vi "gun.vi"() -> ()   [LabVIEW 2011]
uses:
  common/scale_const.ctl
  common/gain_const.ctl
  common/gain_bin_sched_const.ctl
  gun_motor_state.ctl
  <vilib>/Rock Robotics/SystemInterfaces/Typedef/FPGA_TypedefDigitalModule.ctl
  <vilib>/Rock Robotics/SystemInterfaces/DIO/FPGA_DIOChannel.ctl
  signals/Signal.ctl
  <vilib>/Rock Robotics/WPI/Relay/WPI_RelayValue.ctl
  gun_tracking_mode.ctl
  Robot Global Data.vi
  Program Files (x86)/National Instruments/LabVIEW 2011/examples/FRC/I2C/HiTechnic Compass/Driver/HiTechnic Compass.lvlib
panel:
  in  "gun speed const":T1={"min_ana"=0.0, "min_units"=2200.0, "max_ana"=1.0, "max_units"=2200.0}
  in  "fender speed const":T1={"min_ana"=0.0, "min_units"=1650.0, "max_ana"=1.0, "max_units"=1730.0}
  in  "light time":u32=150
  in  "Gains Fender":T2={"Positive"={"kP"=1.4, "kI"=3.3, "kD"=0.06}, "Netative"={"kP"=1.4, "kI"=3.3, "kD"=0.06}}
  in  "Gains Key":T2={"Positive"={"kP"=1.45, "kI"=3.5, "kD"=0.057}, "Netative"={"kP"=1.5, "kI"=3.3, "kD"=0.054}}
  in  "PID Fender":T3={"kP"=1.0, "kI"=3.0, "kD"=0.06}
  in  "interval back key":dbl=1000.0
  in  "interval fender":dbl=1000.0
  in  "interval key":dbl=650.0
  in  "Cam Lock Const":u32=150
  in  "Hood Key":dbl=67.0
  in  "Gun Key":dbl=2200.0
  in  "back key Gun":dbl=2200.0
  in  "back key Hood":dbl=68.0
  in  "Scale Const":T1={"min_ana"=0.0, "min_units"=90.0, "max_ana"=25.5, "max_units"=82.5}
  out "Heading":dbl
  # "Fender Shot"
  # "Key Shot"
  # "Back Key Shot"
  # "kP 1.5\nkI 3.3\nkD .054"
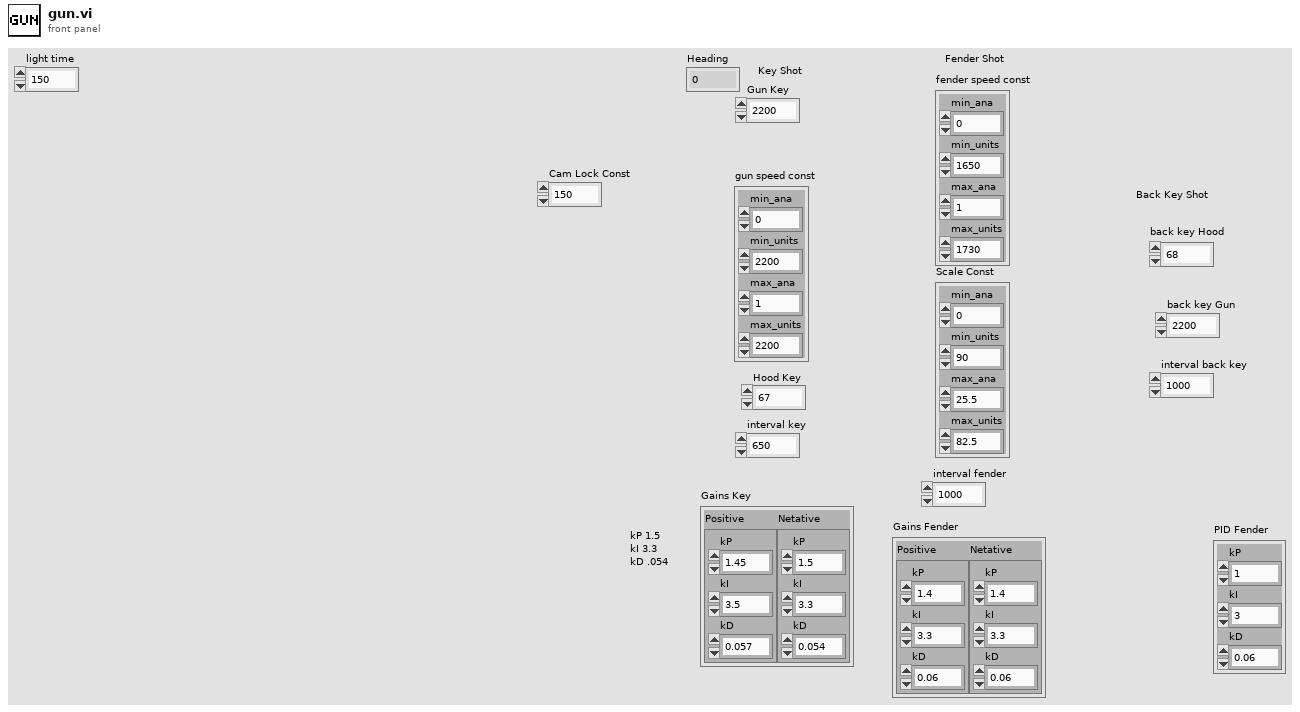
[diagram p1: front panel]
types:
  T1 = typedef "scale_const.ctl" = cluster{"min_ana":dbl, "min_units":dbl, "max_ana":dbl, "max_units":dbl}
  T2 = typedef "gain_bin_sched_const.ctl" = cluster{"Positive":cluster{"kP":dbl, "kI":dbl, "kD":dbl}, "Netative":cluster{"kP":dbl, "kI":dbl, "kD":dbl}}
  T3 = typedef "gain_const.ctl" = cluster{"kP":dbl, "kI":dbl, "kD":dbl}
  T4 = typedef "FPGA_DIOChannel.ctl" = enum8{"DIO 1", "DIO 2", "DIO 3", "DIO 4", "DIO 5", "DIO 6", "DIO 7", "DIO 8", "DIO 9", "DIO 10", "DIO 11", "DIO 12", "DIO 13", "DIO 14", "Invalid"}
  T5 = typedef "FPGA_TypedefDigitalModule.ctl" = enum16{"Digital Module 1", "Digital Module 2"}
  T6 = typedef "gun_motor_state.ctl" = enum16{"Hold Power", "Hold Speed", "Hold Distance", "Stop"}
  T7 = cluster{"Gun Key":dbl, "Shooter Control Mode":T6}
  T8 = typedef "WPI_DigitalInputDevRef.ctl" = cluster{"DevStatus":errorcluster, "DIO Channel":T4, "Digital Module":T5}
  T9 = typedef "WPI_I2CDevRef.ctl" = cluster{"DevStatus":errorcluster, "Digital Module":T5, "Device Address":u8}
  T10 = typedef "WPI_RelayDevRef.ctl" = cluster{"DevStatus":errorcluster, "Relay Channel":T11, "Digital Module":T5, "Relay Direction":T12}
  T11 = typedef "FPGA_DIORelayChannel.ctl" = enum8{"Relay 1", "Relay 2", "Relay 3", "Relay 4", "Relay 5", "Relay 6", "Relay 7", "Relay 8", "Invalid"}
  T12 = typedef "WPI_RelayDirection.ctl" = enum16{"Both directions", "Forward only", "Reverse only"}
  T13 = typedef "Signal.ctl" = enum16{"SIGFIRE", "SIGSTOPSCRIPT", "SIGSTARTGUN", "SIGSTOPGUN", "SIGDISABLED", "SIGENABLED", "SIGUDPTIMEOUT", "SIGNEWVISION_REMOTE", "SIGNEWVISION_LOCAL", "SIGSHOTFIRED", "SIGDOTRACK", "SIGDONTTRACK"}
  T14 = typedef "WPI_RelayValue.ctl" = enum16{"Off", "On", "Forward", "Reverse"}
  T15 = typedef "gun_tracking_mode.ctl" = enum16{"manual_aim", "auto_aim_camera", "preset_center_field", "preset_right_pocket", "preset_left_pocket", "align_center", "align_center_backwards", "auto_aim_key", "align_fold", "auton_custom", "preset_pass", "auto_aim_auton"}
  T16 = typedef "gun_rt_fast_upstream_data.ctl" = cluster{"gun_sensor_speed":dbl, "gun_motor_output":dbl}
  T17 = typedef "gun_rt_slow_upstream_data.ctl" = cluster{"turret":cluster{"turret_analog":dbl, "turret_angle":dbl, "turret_motor":dbl, "turret_idg_state":T18}, "hood":cluster{"hood_analog":dbl, "hood_angle":dbl, "hood_motor":dbl, "hood_idg_state":T18}}
  T18 = typedef "idg_trust_t.ctl" = enum16{"fault_move", "fault_high", "fault_low", "out_high", "out_low", "trust"}
  T19 = typedef "user_data.ctl" = cluster{"Driver":cluster{"Buttons":T20, "Axes":cluster{"L-X":dbl, "L-Y":dbl, "R-X":dbl, "R-Y":dbl, "D-X":dbl, "D-Y":dbl}}, "Operator":cluster{"Buttons":T21, "Axes":cluster{"L-X":dbl, "L-Y":dbl, "Trig":dbl, "R-X":dbl, "R-Y":dbl, "D-X":dbl}}, "Kittys Kat Box":cluster{"Btn1":bool, "Btn2":bool, "Btn3":bool, "LeftKnob":dbl, "RightKnob":dbl, "SW1":bool, "SW2":bool}}
  T20 = typedef "user_buttons_dualaction.ctl" = cluster{"Btn1":bool, "Btn2":bool, "Btn3":bool, "Btn4":bool, "L1":bool, "R1":bool, "L2":bool, "R2":bool, "Face-L":bool, "Face-R":bool, "L3":bool, "R3":bool}
  T21 = typedef "user_buttons_360.ctl" = cluster{"Down":bool, "Right":bool, "Left":bool, "Up":bool, "L1":bool, "R1":bool, "Face-L":bool, "Face-R":bool, "L2":bool, "R2":bool, "Unused":bool, "Unused":bool}
  T22 = typedef "gun_rt_slow_downstream_data.ctl" = cluster{"turret":cluster{"turret_setpoint":dbl, "turret_reset_integral":bool, "turret_manual":dbl, "turret_manual_mode":bool}, "hood":cluster{"hood_setpoint":dbl, "hood_reset_integral":bool, "hood_manual":dbl, "hood_manual_mode":bool}}
  T23 = typedef "gun_preset_pos_t.ctl" = enum16{"Center Field", "Right Pocket", "Left Pocket", "Align Center", "Align Center Backwards", "Fold Side", "Pass"}
  T24 = typedef "gun_preset_bundle_t.ctl" = cluster{"speed":dbl, "turret":dbl, "hood":dbl, "interval":dbl}
  T25 = cluster{"speed":dbl, "hood":dbl, "speed new":dbl}
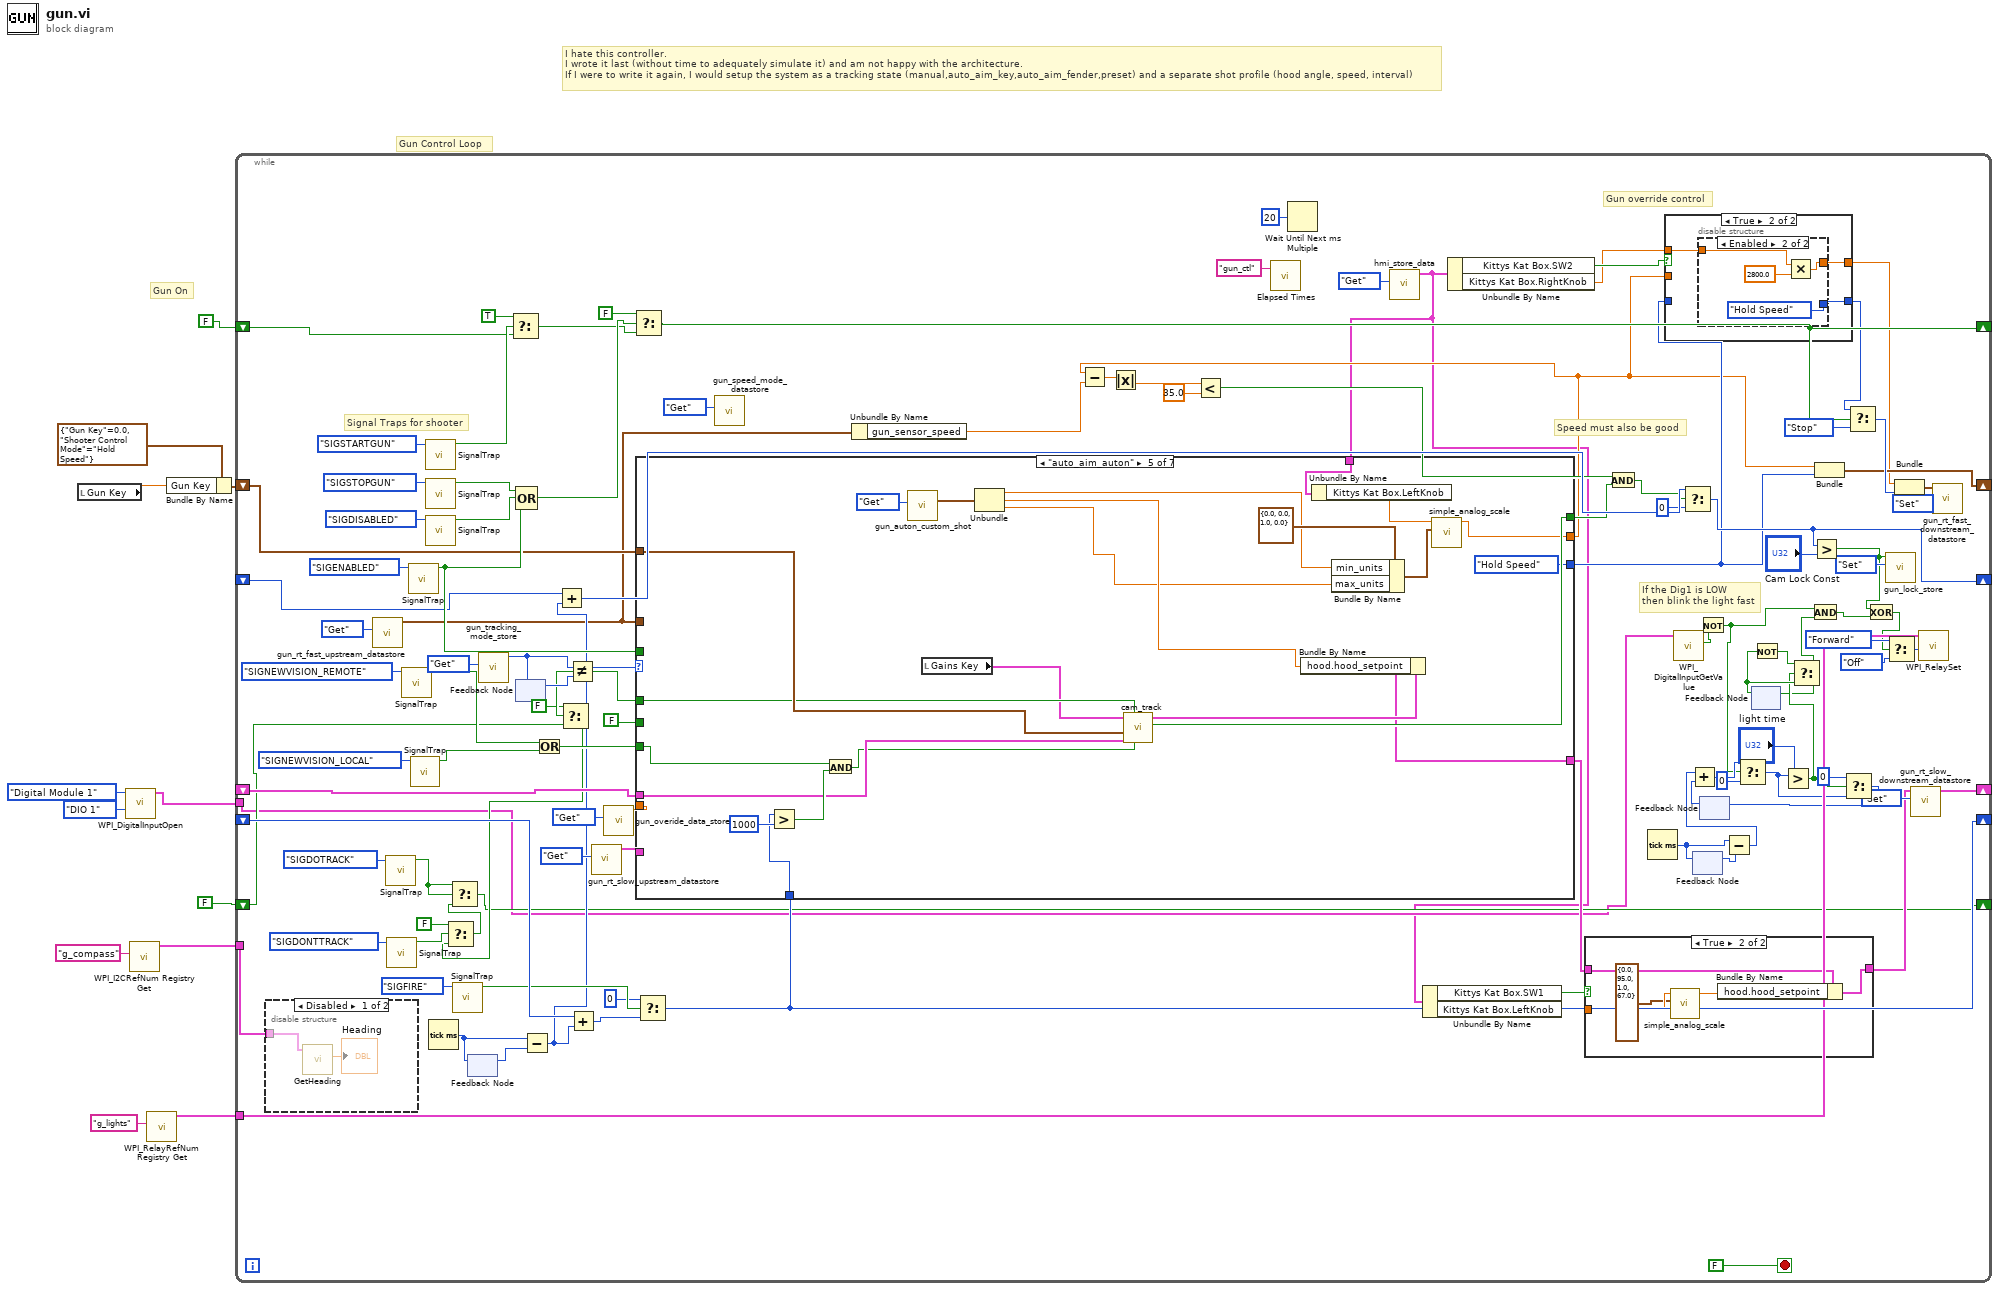
[diagram p0: block diagram]
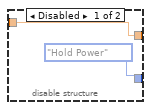
[diagram p4: hidden frame]
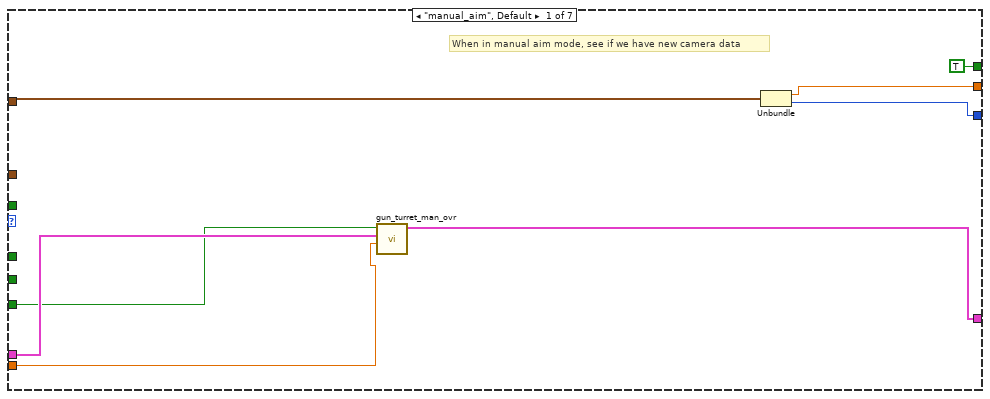
[diagram p6: hidden frame]
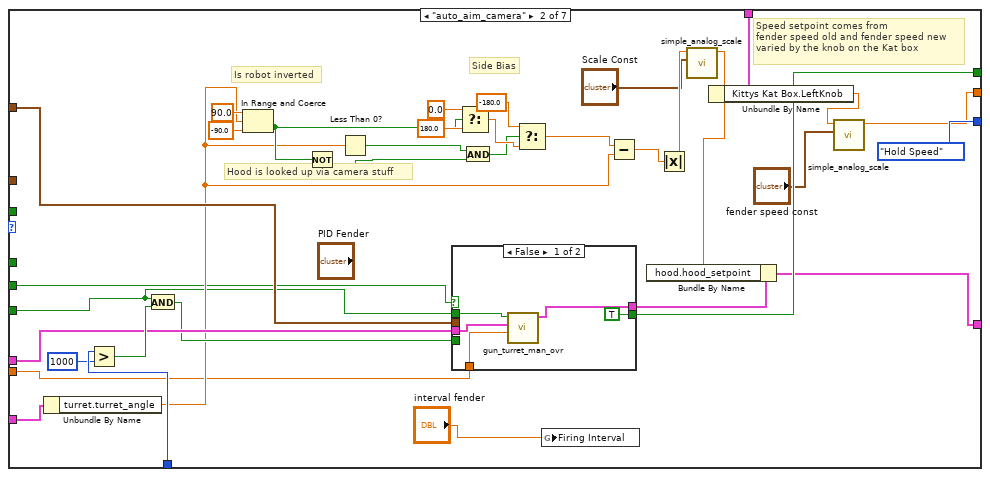
[diagram p7: hidden frame]
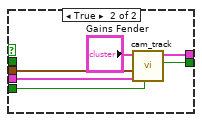
[diagram p8: hidden frame]
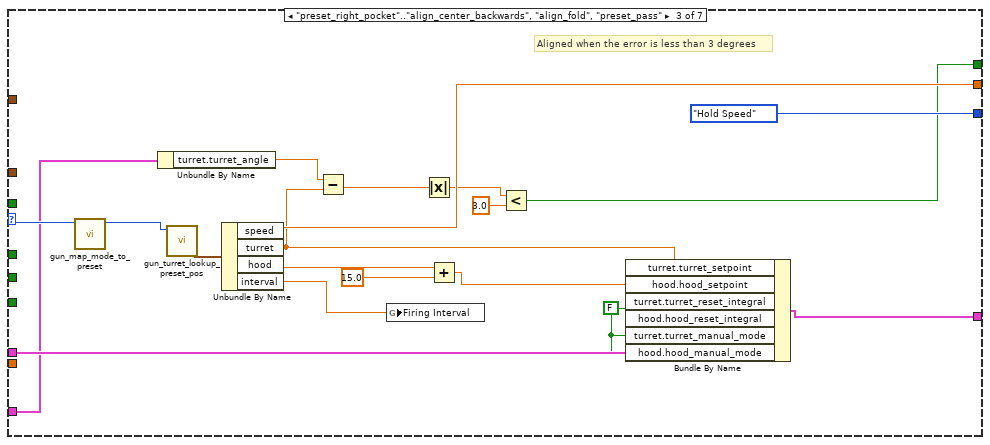
[diagram p9: hidden frame]
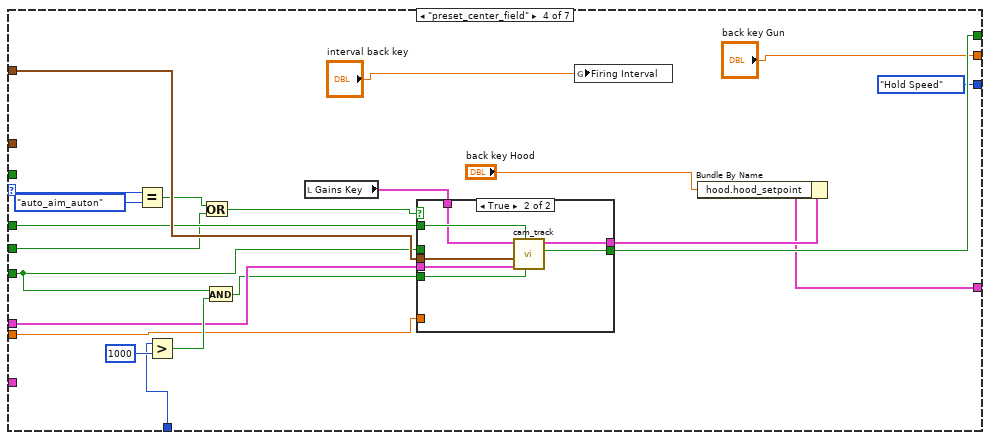
[diagram p10: hidden frame]
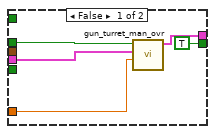
[diagram p11: hidden frame]
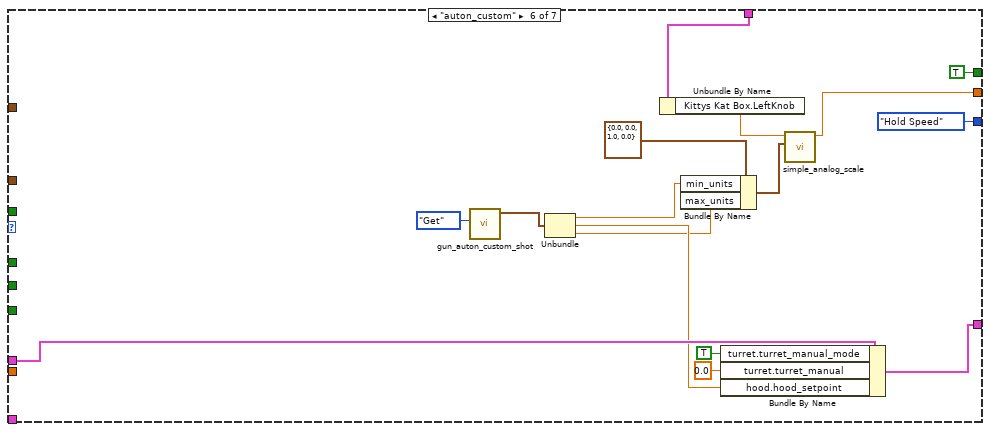
[diagram p12: hidden frame]
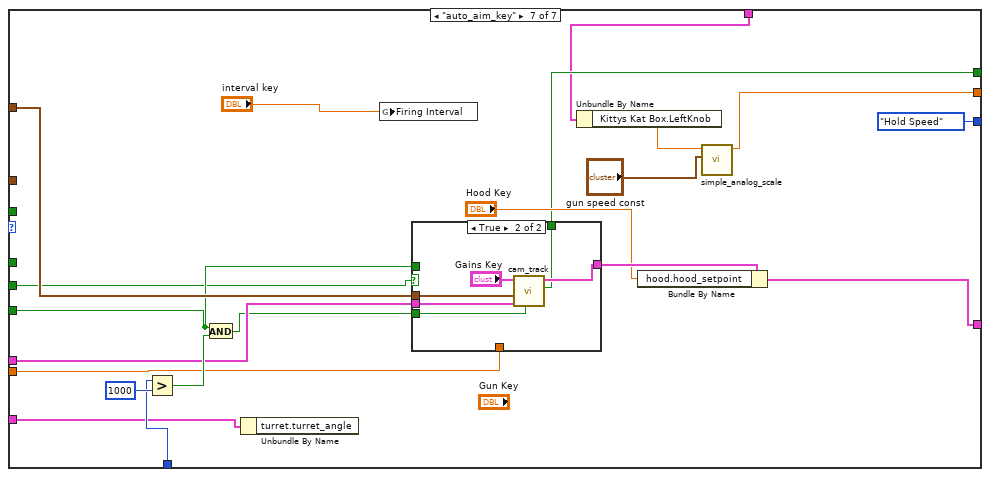
[diagram p13: hidden frame]
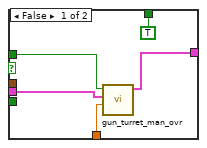
[diagram p14: hidden frame]
diagram:
  # "I hate this controller.\nI wrote it last (without time to adequately simulate it) and am not happy with the architecture.\nIf I were to write it again, I would setup the system as a tracking state (manual,auto_aim_key,auto_aim_fender,preset) and a separate shot profile (hood angle, speed, interval)"
  # "Gun On"
  # "Gun Control Loop"
  n1 = local read "Gun Key"() -> (w5:dbl)
  n2 = call <vilib>:"WPI_DigitalInputOpen.vi"("DIO Channel"=FPGA_DIOChannel."DIO 1", "Digital Module (Module 1)"=FPGA_TypedefDigitalModule."Digital Module 1") -> ("DigitalInputDevRef"=w3:T8)  [unwired: 8 in, 1 out]
  n3 = call <vilib>:"WPI_I2CRefNum Registry Get.vi"("refnum name"="g_compass") -> ("I2CDevRef"=w10:T9)  [unwired: 9 in, 1 out]
  n4 = call <vilib>:"WPI_RelayRefNum Registry Get.vi"("refnum name"="g_lights") -> ("RelayDevRef"=w8:T10)  [unwired: 9 in, 1 out]
  n5 = Bundle By Name(cluster=T7 {"Gun Key"=0.0, "Shooter Control Mode"=enum."Hold Speed"}, "Gun Key"=w5) -> (w6:T7)
  n6 = while {
    shift-right: [w90] -> _
    shift-left: FALSE -> [w120]
    shift-right: [w97] -> _
    shift-left: _ -> [w89]
    shift-right: [w79] -> _
    shift-left: w6 -> [w65]
    tunnel: w10 -> [w88]
    shift-right: [w80] -> _
    shift-left: _ -> [w84]
    shift-right: [w71] -> _
    shift-left: _ -> [w75]
    tunnel: w8 -> [w60]
    shift-right: [w35] -> _
    shift-left: FALSE -> [w36]
    tunnel: w3 -> [w31]
    stop <- FALSE stop-if-true
    # "If the Dig1 is LOW\nthen blink the light fast"
    # "Gun override control"
    # "Speed must also be good"
    # "Signal Traps for shooter"
    n7 = disable-structure shown="Disabled" {
      disable-tunnel: w88 -> [w143 _]
      frame Disabled {
        n8 = call "GetHeading.vi"("I2CDevRef"=w143) -> ("Heading"=→"Heading":dbl)  [unwired: 1 in, 9 out]
      }
      frame Enabled {
      }
    }
    n9 = call "gun_rt_fast_upstream_datastore.vi"("data_store_mode"=enum16{"Set", "Get"}."Get") -> ("gun_rt_fast_upstream_data out"=w64:T16)  [unwired: 10 in]
    n10 = call "SignalTrap.vi"("Signal"=Signal."SIGDOTRACK") -> ("Trapped Signal"=w44:bool)  [unwired: 10 in]
    n11 = call "SignalTrap.vi"("Signal"=Signal."SIGDONTTRACK") -> ("Trapped Signal"=w40:bool)  [unwired: 10 in]
    n12 = call "SignalTrap.vi"("Signal"=Signal."SIGNEWVISION_REMOTE") -> ("Trapped Signal"=w95:bool)  [unwired: 10 in]
    n13 = call "SignalTrap.vi"("Signal"=Signal."SIGENABLED") -> ("Trapped Signal"=w91:bool)  [unwired: 10 in]
    n14 = call "SignalTrap.vi"("Signal"=Signal."SIGNEWVISION_LOCAL") -> ("Trapped Signal"=w94:bool)  [unwired: 10 in]
    n15 = call "SignalTrap.vi"("Signal"=Signal."SIGSTARTGUN") -> ("Trapped Signal"=w121:bool)  [unwired: 10 in]
    n16 = call "SignalTrap.vi"("Signal"=Signal."SIGSTOPGUN") -> ("Trapped Signal"=w118:bool)  [unwired: 10 in]
    n17 = call "SignalTrap.vi"("Signal"=Signal."SIGDISABLED") -> ("Trapped Signal"=w117:bool)  [unwired: 10 in]
    n18 = Tick Count (ms)() -> (millisecond timer value=w85:u32)
    n19 = call "SignalTrap.vi"("Signal"=Signal."SIGFIRE") -> ("Trapped Signal"=w82:bool)  [unwired: 10 in]
    n20 = feedback-in #1(w85) -> ()
    n21 = feedback #1() -> (w86:u32)  [unwired: 1 in]
    n22 = call "gun_tracking_mode_store.vi"("data_store_mode"=enum16{"Set", "Get"}."Get") -> ("gun tracking mode"=w76:T15)  [unwired: 10 in]
    n23 = Select(t=TRUE, s=w121, f=w120) -> (s? t:f=w111:bool)
    n24 = Compound Arithmetic op=OR(w118, w117, w91) -> (w116:bool)
    n25 = feedback-in #2(w76) -> ()
    n26 = feedback #2() -> (w77:T15)  [unwired: 1 in]
    n27 = Subtract(x=w85, y=w86) -> (x-y=w74:u32)
    n28 = Or(x=w95, y=w94) -> (x .or. y?=w93:bool)
    n29 = Add(x=w75, y=w74) -> (x+y=w73:u32)
    n30 = Not Equal?(x=w76, y=w77) -> (x != y?=w43:bool)
    n31 = Select(t=FALSE, s=w43, f=w36) -> (s? t:f=w37:bool)
    n32 = Select(t=FALSE, s=w40, f=w37) -> (s? t:f=w39:bool)
    n33 = Select(t=w44, s=w44, f=w39) -> (s? t:f=w35:bool)
    n34 = Add(x=w84, y=w74) -> (x+y=w83:u32)
    n35 = call "gun_rt_slow_upstream_datastore.vi"("data_store_mode"=enum16{"Set", "Get"}."Get") -> ("gun_rt_slow_upstream_data out"=w92:T17)  [unwired: 10 in]
    n36 = call "gun_overide_data_store.vi"("mode"=enum16{"Set", "Get"}."Get") -> ("Overide Out"=w98:dbl)  [unwired: 10 in]
    n37 = Select(t=FALSE, s=w116, f=w111) -> (s? t:f=w90:bool)
    n38 = Select(t=u32 0, s=w82, f=w83) -> (s? t:f=w80:u32)
    n39 = call "gun_speed_mode_datastore.vi"("data_store_mode"=enum16{"Set", "Get"}."Get") -> ()  [unwired: 10 in, 1 out]
    n40 = Unbundle By Name(w64) -> ("gun_sensor_speed"=w66:dbl)
    n41 = call "Elapsed Times.vi"("Call Name"="gun_ctl") -> ()  [unwired: 2 in, 1 out]
    n42 = Wait Until Next ms Multiple(millisecond multiple=u32 20 ("milliseconds to wait")) -> ()  [unwired: 1 out]
    n43 = call "hmi_store_data.vi"("data_store_mode"=enum16{"Set", "Get"}."Get") -> ("UserData out"=w13:T19)  [unwired: 10 in]
    n44 = case shown="\"auto_aim_auton\"" w76 {
      selector: w76 -> [_ _ w216 w221 _ _ _]
      tunnel: [w146 w154 w213 "back key Gun" w253 w278 w291] -> w51
      tunnel: w98 -> [w148 w156 _ w222 _ _ w295]
      tunnel: w89 -> [w151 w167 w212 w235 w270 w287 w304]
      tunnel: w65 -> [w147 w168 _ w234 w269 _ w303]
      tunnel: w93 -> [w149 w157 _ w223 w261 _ w296]
      tunnel: w92 -> [_ w186 w208 _ _ _ w306]
      tunnel: w91 -> [_ _ _ _ _ _ _]
      tunnel: [w150 w164 w211 w229 w265 w284 w299] -> w48
      tunnel: [w145 gun_motor_state."Hold Speed" ("Shooter Control Mode") gun_motor_state."Hold Speed" ("t") gun_motor_state."Hold Speed" ("Shooter Control Mode") gun_motor_state."Hold Speed" ("Shooter Control Mode") gun_motor_state."Hold Speed" ("Shooter Control Mode") gun_motor_state."Hold Speed" ("Shooter Control Mode")] -> w53
      tunnel: w80 -> [_ w185 _ w236 w271 _ w307]
      tunnel: [TRUE ("Lock") w166 w202 w233 w268 TRUE ("Lock") w298] -> w62
      tunnel: w43 -> [_ _ _ w225 w263 _ _]
      tunnel: w64 -> [_ _ _ _ _ _ _]
      tunnel: FALSE ("t") -> [_ w158 _ w218 _ _ w294]
      tunnel: w13 -> [_ w153 _ _ w254 w279 w292]
      frame "manual_aim", Default {
        # "When in manual aim mode, see if we have new camera data"
        n45 = call "gun_turret_man_ovr.vi"("Overide"=w148, "gun_rt_slow_downstream_data out in"=w151, "Trigger Vision"=w149) -> ("gun_rt_slow_downstream_data out out"=w150:T22)  [unwired: 8 in]
        n46 = Unbundle(w147) -> ("Units"=w146:dbl, "Shooter Control Mode"=w145:T6)
      }
      frame "auto_aim_camera" {
        # "Speed setpoint comes from\nfender speed old and fender speed new\nvaried by the knob on the Kat box"
        # "Side Bias"
        # "Is robot inverted"
        # "Hood is looked up via camera stuff"
        n47 = Unbundle By Name(w186) -> ("turret.turret_angle"=w160:dbl)
        n48 = Greater?(x=w185, y=u32 1000) -> (0:w183:bool)
        n49 = And(x=w157, y=w183) -> (x .and. y?=w161:bool)
        n50 = In Range and Coerce(upper limit=90.0, x=w160, lower limit=-90.0) -> (In Range?=w171:bool)  [unwired: 1 out]
        n51 = Not(x=w171) -> (.not. x?=w172:bool)
        n52 = Less Than 0?(x=w160) -> (x < 0?=w174:bool)
        n53 = case shown="False" w158 {
          tunnel: w168 -> [_ w197]
          tunnel: w167 -> [w190 w196]
          tunnel: [TRUE ("Lock") w195] -> w166
          tunnel: [w189 w194] -> w165
          tunnel: w161 -> [_ w193]
          tunnel: w157 -> [w191 _]
          tunnel: w156 -> [w187 _]
          frame False {
            n54 = call "gun_turret_man_ovr.vi"("Overide"=w187, "gun_rt_slow_downstream_data out in"=w190, "Trigger Vision"=w191) -> ("gun_rt_slow_downstream_data out out"=w189:T22)  [unwired: 8 in]
          }
          frame True {
            n55 = call "cam_track.vi"("Trigger"=w193, "gun_rt_slow_downstream_data out in"=w196, "gun_rt_fast_downstream_data out"=w197, "Gains"="Gains Fender") -> ("Lock"=w195:bool, "gun_rt_slow_downstream_data out out"=w194:T22)  [unwired: 6 in]
          }
        }
        n56 = Select(t=0.0, s=w171, f=180.0) -> (s? t:f=w178:dbl)
        n57 = And(x=w174, y=w172) -> (x .and. y?=w173:bool)
        n58 = Select(t=-180.0, s=w173, f=w178) -> (s? t:f=w176:dbl)
        n59 = global write "Robot Global Data.vi" "Firing Interval"("interval fender") -> ()
        n60 = Subtract(x=w176, y=w160) -> (x-y=w175:dbl)
        n61 = Absolute Value(x=w175) -> (abs(x)=w170:dbl)
        n62 = call "simple_analog_scale.vi"("Scale Const"="Scale Const", "Analog"=w170) -> ("Units"=w163:dbl)  [unwired: 9 in]
        n63 = Bundle By Name(cluster=w165, "hood.hood_setpoint"=w163) -> (w164:T22)
        n64 = Unbundle By Name(w153) -> ("Kittys Kat Box.LeftKnob"=w152:dbl)
        n65 = call "simple_analog_scale.vi"("Scale Const"="fender speed const", "Analog"=w152) -> ("Units"=w154:dbl)  [unwired: 9 in]
      }
      frame "preset_right_pocket".."align_center_backwards", "align_fold", "preset_pass" {
        w210 = FALSE
        # "Aligned when the error is less than 3 degrees"
        n66 = call "gun_map_mode_to_preset.vi"("gun tracking mode"=w216) -> ("Preset Position"=w215:T23)  [unwired: 10 in]
        n67 = Unbundle By Name(w208) -> ("turret.turret_angle"=w207:dbl)
        n68 = call "gun_turret_lookup_preset_pos.vi"("Preset Position"=w215) -> ("Position"=w214:T24)  [unwired: 10 in]
        n69 = Unbundle By Name(w214) -> ("speed"=w213:dbl, "turret"=w206:dbl, "hood"=w201:dbl, "interval"=w198:dbl)
        n70 = Subtract(x=w207, y=w206) -> (x-y=w205:dbl)
        n71 = global write "Robot Global Data.vi" "Firing Interval"(w198) -> ()
        n72 = Absolute Value(x=w205) -> (abs(x)=w204:dbl)
        n73 = Add(x=w201, y=15.0) -> (x+y=w200:dbl)
        n74 = Less?(x=w204, y=3.0) -> (x < y?=w202:bool)
        n75 = Bundle By Name(cluster=w212, "turret.turret_setpoint"=w206, "hood.hood_setpoint"=w200, "turret.turret_reset_integral"=w210, "hood.hood_reset_integral"=w210, "turret.turret_manual_mode"=w210, "hood.hood_manual_mode"=w210) -> (w211:T22)
      }
      frame "preset_center_field" {
        n76 = Equal?(x=w221, y=gun_tracking_mode."auto_aim_auton") -> (x = y?=w219:bool)
        n77 = Greater?(x=w236, y=u32 1000) -> (0:w237:bool)
        n78 = Or(x=w219, y=w218) -> (x .or. y?=w217:bool)
        n79 = And(x=w223, y=w237) -> (x .and. y?=w227:bool)
        n80 = local read "Gains Key"() -> (w224:T2)
        n81 = case shown="True" w217 {
          tunnel: w235 -> [w242 w250]
          tunnel: w234 -> [_ w249]
          tunnel: [TRUE ("Lock") w248] -> w233
          tunnel: [w241 w247] -> w230
          tunnel: w227 -> [_ w246]
          tunnel: w225 -> [_ w245]
          tunnel: w224 -> [_ w244]
          tunnel: w223 -> [w243 _]
          tunnel: w222 -> [w239 _]
          frame False {
            n82 = call "gun_turret_man_ovr.vi"("Overide"=w239, "gun_rt_slow_downstream_data out in"=w242, "Trigger Vision"=w243) -> ("gun_rt_slow_downstream_data out out"=w241:T22)  [unwired: 8 in]
          }
          frame True {
            n83 = call "cam_track.vi"("Trigger"=w246, "state change"=w245, "gun_rt_slow_downstream_data out in"=w250, "gun_rt_fast_downstream_data out"=w249, "Gains"=w244) -> ("Lock"=w248:bool, "gun_rt_slow_downstream_data out out"=w247:T22)  [unwired: 5 in]
          }
        }
        n84 = global write "Robot Global Data.vi" "Firing Interval"("interval back key") -> ()
        n85 = Bundle By Name(cluster=w230, "hood.hood_setpoint"="back key Hood") -> (w229:T22)
      }
      frame "auto_aim_auton" {
        n86 = Greater?(x=w271, y=u32 1000) -> (0:w272:bool)
        n87 = And(x=w261, y=w272) -> (x .and. y?=w264:bool)
        n88 = call "gun_auton_custom_shot.vi"("data_store_mode"=enum16{"Set", "Get"}."Get") -> ("shot params out"=w259:T25)  [unwired: 10 in]
        n89 = local read "Gains Key"() -> (w262:T2)
        n90 = Unbundle(w259) -> ("speed"=w252:dbl, "hood"=w258:dbl, "speed new"=w251:dbl)
        n91 = call "cam_track.vi"("Trigger"=w264, "state change"=w263, "gun_rt_slow_downstream_data out in"=w270, "gun_rt_fast_downstream_data out"=w269, "Gains"=w262) -> ("Lock"=w268:bool, "gun_rt_slow_downstream_data out out"=w266:T22)  [unwired: 5 in]
        n92 = Bundle By Name(cluster=w266, "hood.hood_setpoint"=w258) -> (w265:T22)
        n93 = Unbundle By Name(w254) -> ("Kittys Kat Box.LeftKnob"=w257:dbl)
        n94 = Bundle By Name(cluster=T1 {"min_ana"=0.0, "min_units"=0.0, "max_ana"=1.0, "max_units"=0.0} ("Scale Const"), "min_units"=w252, "max_units"=w251) -> (w255:T1)
        n95 = call "simple_analog_scale.vi"("Scale Const"=w255, "Analog"=w257) -> ("Units"=w253:dbl)  [unwired: 9 in]
      }
      frame "auton_custom" {
        n96 = call "gun_auton_custom_shot.vi"("data_store_mode"=enum16{"Set", "Get"}."Get") -> ("shot params out"=w282:T25)  [unwired: 10 in]
        n97 = Unbundle(w282) -> ("speed"=w275:dbl, "hood"=w281:dbl, "speed new"=w274:dbl)
        n98 = Unbundle By Name(w279) -> ("Kittys Kat Box.LeftKnob"=w280:dbl)
        n99 = Bundle By Name(cluster=T1 {"min_ana"=0.0, "min_units"=0.0, "max_ana"=1.0, "max_units"=0.0} ("Scale Const"), "min_units"=w275, "max_units"=w274) -> (w276:T1)
        n100 = Bundle By Name(cluster=w287, "turret.turret_manual_mode"=TRUE, "turret.turret_manual"=0.0, "hood.hood_setpoint"=w281) -> (w284:T22)
        n101 = call "simple_analog_scale.vi"("Scale Const"=w276, "Analog"=w280) -> ("Units"=w278:dbl)  [unwired: 9 in]
      }
      frame "auto_aim_key" {
        n102 = Greater?(x=w307, y=u32 1000) -> (0:w308:bool)
        n103 = And(x=w296, y=w308) -> (x .and. y?=w302:bool)
        n104 = Unbundle By Name(w306) -> ()  [unwired: 1 out]
        n105 = global write "Robot Global Data.vi" "Firing Interval"("interval key") -> ()
        n106 = case shown="True" w294 {
          tunnel: w304 -> [w312 w320]
          tunnel: w303 -> [_ w319]
          tunnel: w302 -> [_ w318]
          tunnel: [w314 w317] -> w301
          tunnel: [TRUE ("Lock") w316] -> w298
          tunnel: w296 -> [w311 _]
          tunnel: w295 -> [w310 _]
          frame False {
            n107 = call "gun_turret_man_ovr.vi"("Overide"=w310, "gun_rt_slow_downstream_data out in"=w312, "Trigger Vision"=w311) -> ("gun_rt_slow_downstream_data out out"=w314:T22)  [unwired: 8 in]
          }
          frame True {
            n108 = call "cam_track.vi"("Trigger"=w318, "gun_rt_slow_downstream_data out in"=w320, "gun_rt_fast_downstream_data out"=w319, "Gains"="Gains Key") -> ("Lock"=w316:bool, "gun_rt_slow_downstream_data out out"=w317:T22)  [unwired: 6 in]
          }
        }
        n109 = Unbundle By Name(w292) -> ("Kittys Kat Box.LeftKnob"=w293:dbl)
        n110 = Bundle By Name(cluster=w301, "hood.hood_setpoint"="Hood Key") -> (w299:T22)
        n111 = call "simple_analog_scale.vi"("Scale Const"="gun speed const", "Analog"=w293) -> ("Units"=w291:dbl)  [unwired: 9 in]
      }
    }
    n112 = Subtract(x=w51, y=w66) -> (x-y=w67:dbl)
    n113 = Absolute Value(x=w67) -> (abs(x)=w68:dbl)
    n114 = Less?(x=w68, y=35.0) -> (x < y?=w63:bool)
    n115 = Unbundle By Name(w13) -> ("Kittys Kat Box.SW1"=w49:bool, "Kittys Kat Box.LeftKnob"=w46:dbl)
    n116 = Unbundle By Name(w13) -> ("Kittys Kat Box.SW2"=w55:bool, "Kittys Kat Box.RightKnob"=w50:dbl)
    n117 = case shown="True" w49 {
      tunnel: w48 -> [w125 w130]
      tunnel: [w125 w129] -> w47
      tunnel: w46 -> [_ w127]
      frame False {
      }
      frame True {
        n118 = call "simple_analog_scale.vi"("Scale Const"=T1 {"min_ana"=0.0, "min_units"=95.0, "max_ana"=1.0, "max_units"=67.0}, "Analog"=w127) -> ("Units"=w128:dbl)  [unwired: 9 in]
        n119 = Bundle By Name(cluster=w130, "hood.hood_setpoint"=w128) -> (w129:T22)
      }
    }
    n120 = And(x=w63, y=w62) -> (x .and. y?=w61:bool)
    n121 = Tick Count (ms)() -> (millisecond timer value=w30:u32)
    n122 = case shown="True" w55 {
      tunnel: [w132 w135] -> w54
      tunnel: w53 -> [w132 _]
      tunnel: [w131 w134] -> w52
      tunnel: w51 -> [w131 _]
      tunnel: w50 -> [_ w133]
      frame False {
      }
      frame True {
        n123 = disable-structure shown="Enabled" {
          disable-tunnel: [gun_motor_state."Hold Power" ("Shooter Control Mode") gun_motor_state."Hold Speed" ("Shooter Control Mode")] -> w135
          disable-tunnel: [w136 w139] -> w134
          disable-tunnel: w133 -> [w136 w140]
          frame Disabled {
          }
          frame Enabled {
            n124 = Multiply(x=w140, y=2800.0) -> (x*y=w139:dbl)
          }
        }
      }
    }
    n125 = call <vilib>:"WPI_DigitalInputGetValue.vi"("DigitalInputDevRef"=w31) -> ("Value"=w14:bool)  [unwired: 8 in, 2 out]
    n126 = Select(t=w73, s=w61, f=u32 0) -> (s? t:f=w71:u32)
    n127 = feedback-in #3(w30) -> ()
    n128 = feedback #3() -> (w29:u32)  [unwired: 1 in]
    n129 = Not(x=w14) -> (.not. x?=w15:bool)
    n130 = feedback #4() -> (w28:u32)  [unwired: 1 in]
    n131 = Subtract(x=w30, y=w29) -> (x-y=w26:u32)
    n132 = Add(x=w26, y=w28) -> (x+y=w27:u32)
    n133 = Select(t=w27, s=w15, f=u32 0) -> (s? t:f=w23:u32)
    n134 = feedback #5() -> (w19:bool)  [unwired: 1 in]
    n135 = Not(x=w19) -> (.not. x?=w20:bool)
    n136 = Greater?(x=w23, y="light time") -> (0:w18:bool)
    n137 = Select(t=w20, s=w18, f=w19) -> (s? t:f=w17:bool)
    n138 = feedback-in #5(w17) -> ()
    n139 = And(x=w15, y=w17) -> (x .and. y?=w16:bool)
    n140 = Greater?(x=w71, y="Cam Lock Const") -> (0:w32:bool)
    n141 = Bundle("Units"=w51, "Shooter Control Mode"=w53) -> (w79:cluster{"Units":dbl, "Shooter Control Mode":T6})  [unwired: 1 in]
    n142 = Select(t=u32 0, s=w18, f=w23) -> (s? t:f=w22:u32)
    n143 = feedback-in #4(w22) -> ()
    n144 = Select(t=w54, s=w90, f=gun_motor_state."Stop") -> (s? t:f=w109:T6)
    n145 = Exclusive Or(1:w16, 2:w32) -> (0:w33:bool)
    n146 = call "gun_lock_store.vi"("data_store_mode"=enum16{"Set", "Get"}."Set", "Lock"=w32) -> ()  [unwired: 9 in, 1 out]
    n147 = Select(t=WPI_RelayValue."Forward", s=w33, f=WPI_RelayValue."Off" ("RelayValue")) -> (s? t:f=w58:T14)
    n148 = Bundle("Units"=w52, "f"=w109) -> (w96:cluster{"Units":dbl, "f":T6})  [unwired: 1 in]
    n149 = call "gun_rt_slow_downstream_datastore.vi"("data_store_mode"=enum16{"Set", "Get"}."Set", "gun_rt_slow_downstream_data"=w47) -> ("gun_rt_slow_downstream_data out"=w97:T22)  [unwired: 9 in]
    n150 = call <vilib>:"WPI_RelaySet.vi"("RelayValue"=w58, "RelayDevRef"=w60) -> ()  [unwired: 8 in, 2 out]
    n151 = call "gun_rt_fast_downstream_datastore.vi"("data_store_mode"=enum16{"Set", "Get"}."Set", "gun_rt_fast_downstream_data"=w96) -> ()  [unwired: 9 in, 1 out]
  }
